vi "Read channelType_spectrum.vi"(8 "error in (no error)":errorcluster, 11 "OSA300 in":refnum<class "OSA300.lvclass">) -> (0 "error out":errorcluster, 2 "channelType_spectrum":T1, 3 "OSA300 out":refnum<class "OSA300.lvclass">)   [LabVIEW 2010, in "OSA300.lvclass"]
uses:
  OSA300.lvclass
  _misc/Thorlabs_FTS_misc.llb/channelType_spectrum.ctl
  OSA20X_misc.lvlib
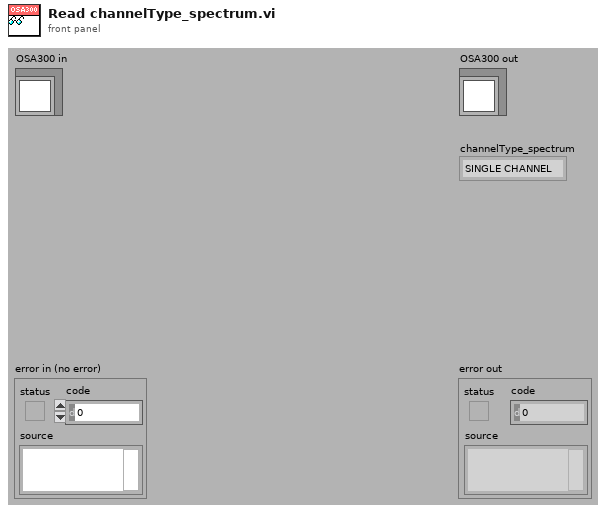
[diagram p1: front panel]
types:
  T1 = typedef "OSA20X_misc.lvlib/channelType_spectrum.ctl" = enum16{"SINGLE CHANNEL", "STICHED"}
  T2 = typedef "OSA300.lvclass/OSA300_DVR.ctl" = refnum<data-value>
  T3 = typedef "OSA300.lvclass/OSA300_data.ctl" = cluster{"channel DUT":refnum<class "OSAchannel.lvclass">[], "channelType_spectrum":T1, "channel REF nr":i32, "channel stiched":u32, "channel DUT (index)":i32, "channel nr":i32, "Ref":u32}
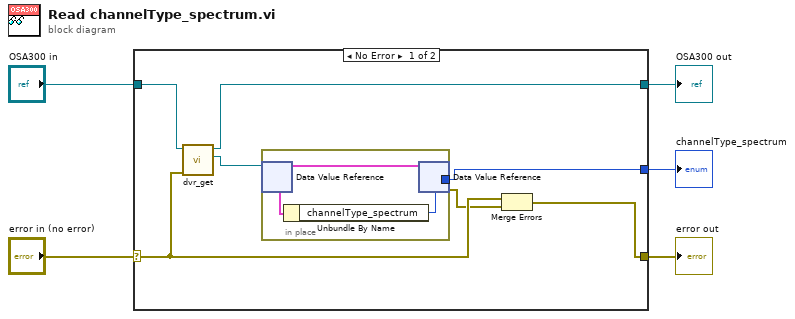
[diagram p0: block diagram]
diagram:
  n1 = case shown="No Error" "error in (no error)" {
    selector: "error in (no error)" -> [w9 w15]
    tunnel: [w7 w15] -> w4
    tunnel: [w10 w16] -> w2
    tunnel: "OSA300 in" -> [w11 w16]
    tunnel: [w6 _] -> w1
    frame No Error {
      n2 = call "dvr_get.vi"("error in (no error)"=w9, "OSA300 in"=w11) -> ("data value ref"=w12:T2, "OSA300 out"=w10:refnum<class "OSA300.lvclass">)  [unwired: 7 in, 1 out]
      n3 = in-place {
        in-place-border: [w13] -> w6
        n4 = in-place-dvr #1(w12) -> (w14:T3)  [unwired: 1 out]
        n5 = Unbundle By Name(w14) -> ("channelType_spectrum"=w13:T1)
        n6 = in-place-dvr #1(w14) -> (w8:errorcluster)  [unwired: 1 out]
      }
      n7 = Merge Errors(w9, w8) -> (w7:errorcluster)
    }
    frame Error {
    }
  }
  "error out" <- w4
  "OSA300 out" <- w2
  "channelType_spectrum" <- w1
